vi "Queue Command.vi"(8 "millisecond timer value":u32, 10 "Array in":T1(array[cluster]), 11 "Queue in":refnum<queue>) -> (2 "Array out":T1(array[cluster]), 3 "error out":errorcluster)   [LabVIEW 2025]
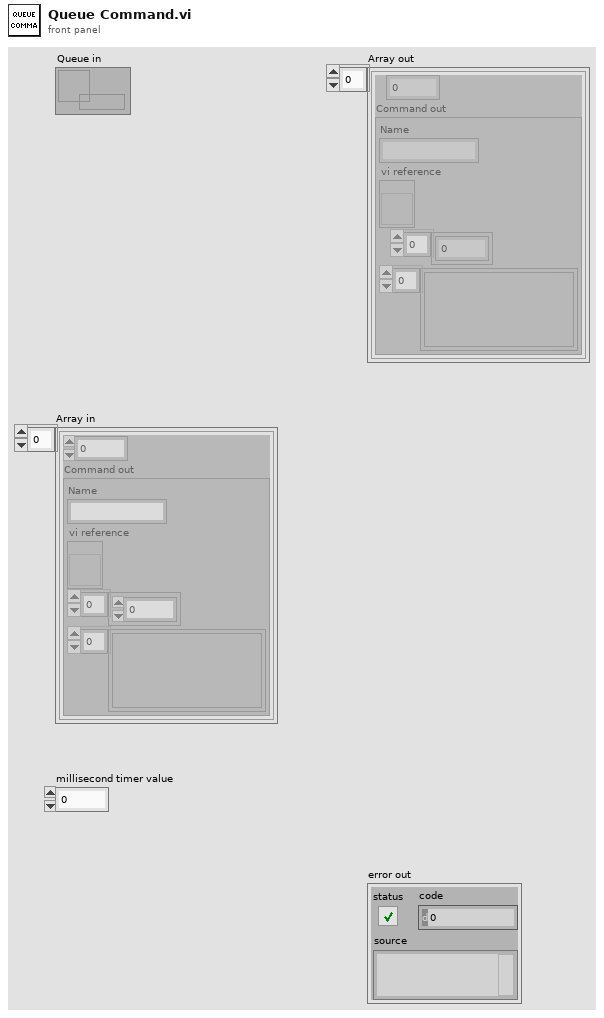
[diagram p1: front panel]
types:
  T1 = cluster{dbl, "Command out":cluster{"Name":string, "vi reference":refnum<vi>, i32[], variant[]}}[]
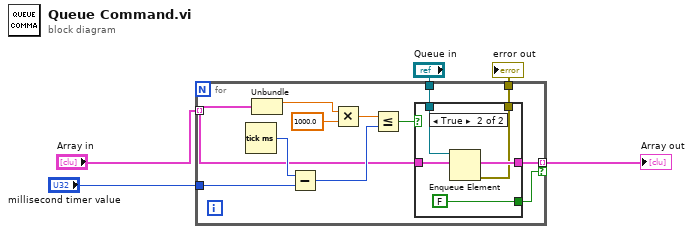
[diagram p0: block diagram]
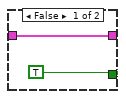
[diagram p2: hidden frame]
diagram:
  n1 = for {
    tunnel: "millisecond timer value" -> [w16]
    tunnel: "Queue in" -> [w10]
    tunnel: "Array in" -> [w7] mode=indexing
    tunnel: [w9] -> w3 mode=indexing if=w8
    tunnel: [w6] -> w5
    n2 = Tick Count (ms)() -> (millisecond timer value=w17:u32)
    n3 = Unbundle(w7) -> (w15:dbl)  [unwired: 1 out]
    n4 = Subtract(x=w17, y=w16) -> (x-y=w12:u32)
    n5 = Multiply(x=w15, y=1000.0) -> (x*y=w13:dbl)
    n6 = Less Or Equal?(x=w13, y=w12) -> (x <= y?=w11:bool)
    n7 = case shown="True" w11 {
      tunnel: w10 -> [_ w23]
      tunnel: w7 -> [w18 w22]
      tunnel: [w18 w22] -> w9
      tunnel: [TRUE FALSE] -> w8
      tunnel: [_ w20] -> w6
      frame False {
      }
      frame True {
        n8 = Enqueue Element(queue=w23, element=w22) -> (error out=w20:errorcluster)  [unwired: 2 in, 2 out]
      }
    }
  }
  "error out" <- w5
  "Array out" <- w3
